vi "Create Cell Range.vi"(8 "error in":errorcluster, 11 "Cell Range":string) -> (0 "error out":errorcluster, 3 "Cell Range":string[][](array[string]))   [LabVIEW 2019, in "Open Xml.lvlib"]
uses:
  Open Xml.lvlib
  <vilib>/Analysis/1siggen.llb/Ramp Pattern by Delta.vi
  <vilib>/Analysis/NI_AALBase.lvlib
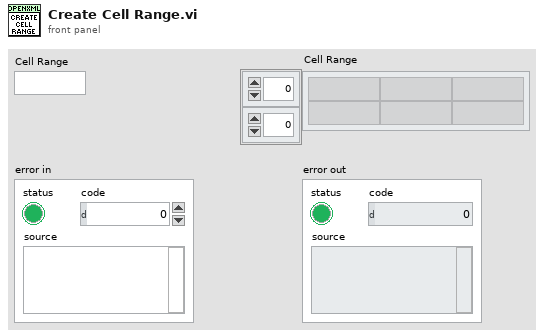
[diagram p1: front panel]
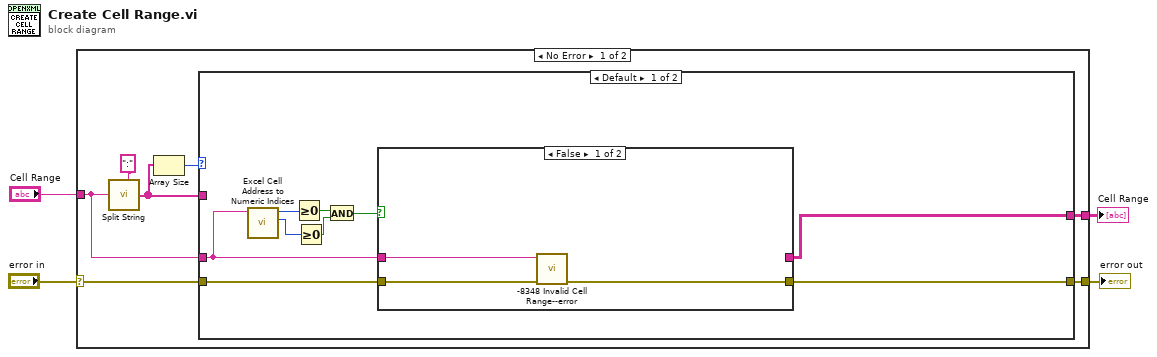
[diagram p0: block diagram]
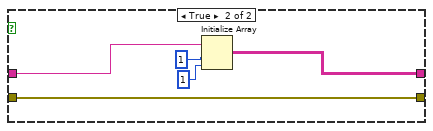
[diagram p2: hidden frame]
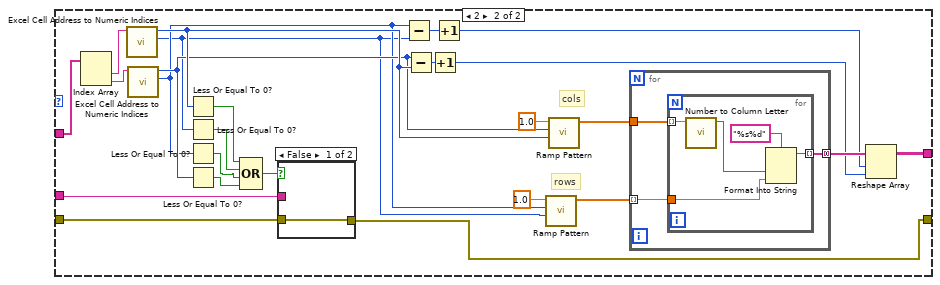
[diagram p3: hidden frame]
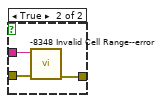
[diagram p4: hidden frame]
diagram:
  n1 = case shown="No Error" "error in" {
    selector: "error in" -> [w8 w66]
    tunnel: [w7 w66] -> w3
    tunnel: "Cell Range" -> [w6 _]
    tunnel: [w5 _] -> w1
    frame No Error {
      n2 = call <vilib>:"Split String.vi"("Split Pattern"=":", "Input String"=w6) -> ("Split String"=w10:string[])  [unwired: 5 in]
      n3 = Array Size(array=w10) -> (size(s)=w9:i32)
      n4 = case shown="Default" w9 {
        tunnel: w10 -> [_ w48]
        tunnel: w8 -> [w15 w39]
        tunnel: [w14 w29] -> w7
        tunnel: w6 -> [w13 w35]
        tunnel: [w12 w45] -> w5
        frame Default {
          n5 = call "Excel Cell Address to Numeric Indices.vi"("Cell Name"=w13) -> ("Row Number"=w16:i32, "Column Number"=w20:i32)  [unwired: 9 in]
          n6 = Greater Or Equal To 0?(x=w20) -> (x >= 0?=w19:bool)
          n7 = Greater Or Equal To 0?(x=w16) -> (x >= 0?=w18:bool)
          n8 = And(x=w19, y=w18) -> (x .and. y?=w17:bool)
          n9 = case shown="False" w17 {
            tunnel: w15 -> [w23 w28]
            tunnel: [w22 w28] -> w14
            tunnel: w13 -> [w21 w27]
            tunnel: [_ w26] -> w12
            frame False {
              n10 = call "-8348 Invalid Cell Range--error.vi"("error in"=w23, "Argument"=w21) -> ("error out"=w22:errorcluster)  [unwired: 9 in]
            }
            frame True {
              n11 = Initialize Array(w27, 1 ("dimension size"), 1 ("dimension size")) -> (w26:string[][])
            }
          }
        }
        frame 2 {
          # "rows"
          # "cols"
          n12 = Index Array(array=w48) -> (element #1=w47:string, element #2=w46:string)  [unwired: 2 in]
          n13 = call "Excel Cell Address to Numeric Indices.vi"("Cell Name"=w47) -> ("Row Number"=w30:i32, "Column Number"=w33:i32)  [unwired: 9 in]
          n14 = call "Excel Cell Address to Numeric Indices.vi"("Cell Name"=w46) -> ("Row Number"=w31:i32, "Column Number"=w32:i32)  [unwired: 9 in]
          n15 = Less Or Equal To 0?(x=w33) -> (x <= 0?=w36:bool)
          n16 = Less Or Equal To 0?(x=w30) -> (x <= 0?=w37:bool)
          n17 = Less Or Equal To 0?(x=w31) -> (x <= 0?=w38:bool)
          n18 = Less Or Equal To 0?(x=w32) -> (x <= 0?=w40:bool)
          n19 = Compound Arithmetic op=OR(w36, w37, w38, w40) -> (w34:bool)
          n20 = case shown="False" w34 {
            tunnel: w39 -> [w54 w57]
            tunnel: w35 -> [_ w56]
            tunnel: [w54 w55] -> w29
            frame False {
            }
            frame True {
              n21 = call "-8348 Invalid Cell Range--error.vi"("error in"=w57, "Argument"=w56) -> ("error out"=w55:errorcluster)  [unwired: 9 in]
            }
          }
          n22 = Subtract(x=w31, y=w30) -> (x-y=w44:i32)
          n23 = Subtract(x=w32, y=w33) -> (x-y=w43:i32)
          n24 = Increment(x=w43) -> (x+1=w41:i32)
          n25 = Increment(x=w44) -> (x+1=w42:i32)
          n26 = call-poly <vilib>:"Ramp Pattern.vi"("start"=w30, "end"=w31, "delta"=1.0) -> ("Ramp Pattern"=w49:dbl[])  [unwired: 6 in, 2 out]
          n27 = call-poly <vilib>:"Ramp Pattern.vi"("start"=w33, "end"=w32, "delta"=1.0) -> ("Ramp Pattern"=w50:dbl[])  [unwired: 6 in, 2 out]
          n28 = for {
            tunnel: [w59] -> w53 mode=concatenating
            tunnel: w50 -> [w58]
            tunnel: w49 -> [w60] mode=indexing
            n29 = for {
              tunnel: w60 -> [w64]
              tunnel: [w63] -> w59 mode=indexing
              tunnel: w58 -> [w62] mode=indexing
              n30 = call "Number to Column Letter.vi"("Number"=w62) -> ("Letter"=w61:string)  [unwired: 10 in]
              n31 = Format Into String(format string="%s%d", w61, w64) -> (resulting string=w63:string)  [unwired: 2 in, 1 out]
            }
          }
          n32 = Reshape Array(w53, w42, w41) -> (w45:string[][])
        }
      }
    }
    frame Error {
    }
  }
  "error out" <- w3
  "Cell Range" <- w1
